vi "FTW-ProjectItem-IDtoRef.vi"(0 "Project Ref":refnum<vi>, 5 "Item ID":string, 11 "error in":errorcluster) -> (4 "Project Ref out":refnum<vi>, 6 "ProjectItem Ref":refnum<vi>, 8 "Display Name":string, 10 "Item Type GUID":string, 15 "error out":errorcluster)   [LabVIEW 2012]
panel:
  # "Inputs"
  # "Outputs"
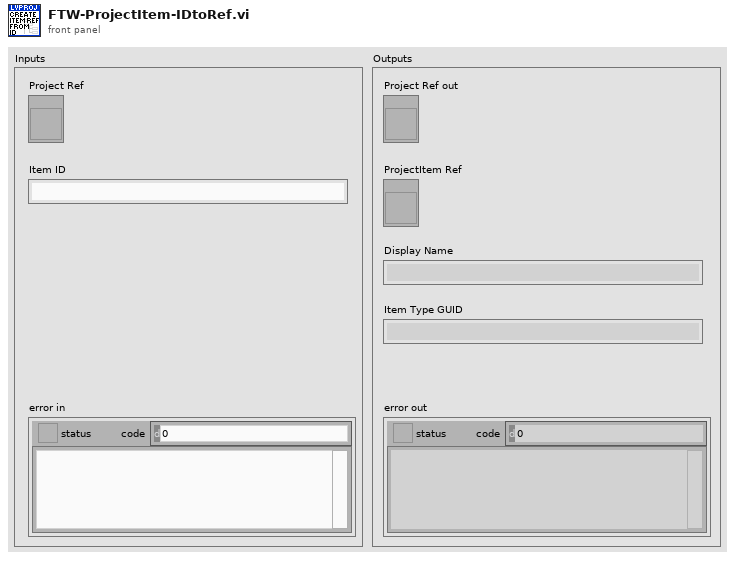
[diagram p1: front panel]
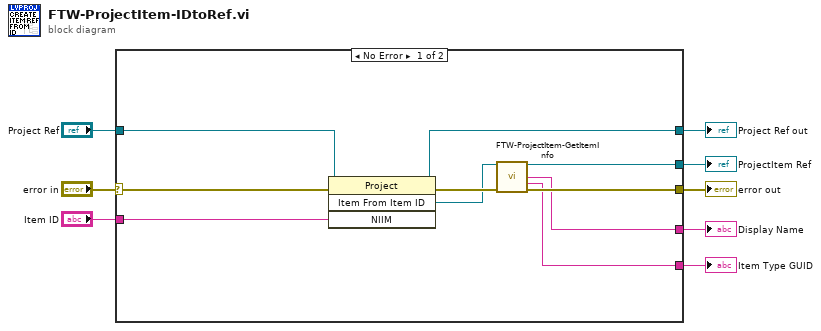
[diagram p0: block diagram]
diagram:
  n1 = case shown="No Error" "error in" {
    selector: "error in" -> [w18 w20]
    tunnel: [w15 w20] -> w8
    tunnel: "Item ID" -> [w17 _]
    tunnel: [w13 _] -> w5
    tunnel: [w12 _] -> w4
    tunnel: [w11 _] -> w3
    tunnel: "Project Ref" -> [w10 w19]
    tunnel: [w9 w19] -> w1
    frame No Error {
      n2 = invoke class="Project" method="Item From Item ID"(reference=w10, error in=w18, "NIIM"=w17) -> (reference out=w9:refnum<vi>, error out=w16:errorcluster, "GetItemFromNIIM"=w14:refnum<vi>)  [unwired: 1 in, 1 out]
      n3 = call "FTW-ProjectItem-GetItemInfo.vi"("ProjectItem"=w14, "error in"=w16) -> ("ProjectItem out"=w13:refnum<vi>, "Display Name"=w12:string, "Item Type GUID"=w11:string, "error out"=w15:errorcluster)  [unwired: 9 in, 1 out]
    }
    frame Error {
    }
  }
  "error out" <- w8
  "ProjectItem Ref" <- w5
  "Display Name" <- w4
  "Item Type GUID" <- w3
  "Project Ref out" <- w1
